vi "Set DDG External Output Step Enabled.vi"(10 "uiEnabled":u32, 11 "uiIndex":u32) -> (3 "function return":u32)   [LabVIEW 2018, in "Copy of Andor SDK.lvlib"]
doc: "EXPNETTYPE unsigned int WINAPI SetDDGExternalOutputStepEnabled(at_u32 uiIndex, at_u32 uiEnabled);"
uses:
  Copy of Andor SDK.lvlib
  <userlib>/Andor SDK/ATMCD32D.dll
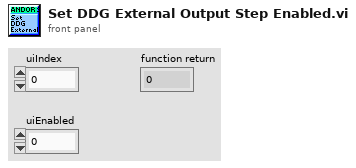
[diagram p1: front panel]
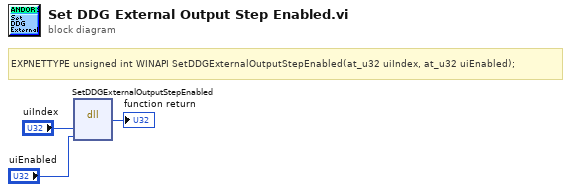
[diagram p0: block diagram]
diagram:
  # "EXPNETTYPE unsigned int WINAPI SetDDGExternalOutputStepEnabled(at_u32 uiIndex, at_u32 uiEnabled);"
  n1 = dll-call lib="C:/Program Files (x86)/National Instruments/LabVIEW 2018/user.lib/Andor SDK/ATMCD32D.*" fn="SetDDGExternalOutputStepEnabled"("uiIndex"="uiIndex", "uiEnabled"="uiEnabled") -> (→"function return":u32)  [unwired: 5 in, 2 out]
